vi "FTW-Subscription-Destroy.vi"(0 "FTW Subscription":refnum<class "FTW-Subscription.lvclass">, 11 "error in":errorcluster) -> (15 "error out":errorcluster)   [LabVIEW 2013, in "FTW-Subscription.lvclass"]
uses:
  FTW-Subscription.lvclass
  FTW-Subscription.lvclass/FTW-Subscription.ctl
  socket/FTW-Socket.lvclass
panel:
  # "Inputs"
  # "Outputs"
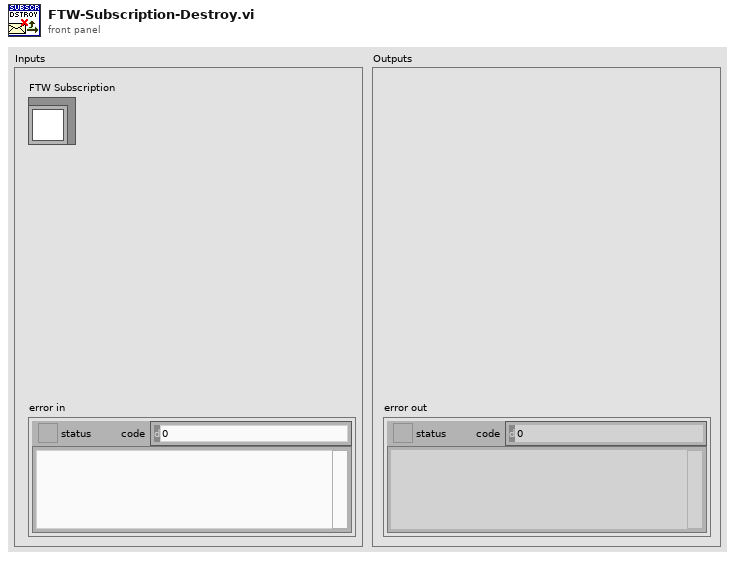
[diagram p1: front panel]
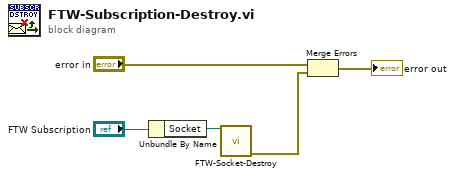
[diagram p0: block diagram]
diagram:
  n1 = Unbundle By Name("FTW Subscription") -> ("Socket"=w1:refnum<class "FTW-Socket.lvclass">)
  n2 = call-dynamic "FTW-Socket-Destroy.vi"("FTW Socket"=w1) -> ("error out"=w2:errorcluster)  [unwired: 14 in]
  n3 = Merge Errors("error in", w2) -> (→"error out":errorcluster)
